vi "Edit Warning.vi"(7 "Warning in":string) -> (3 "Warning out":string)   [LabVIEW 2021, in "Converter.lvlib"]
uses:
  Converter.lvlib
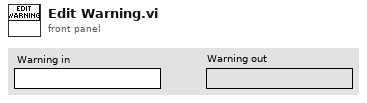
[diagram p1: front panel]
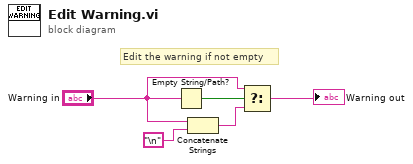
[diagram p0: block diagram]
diagram:
  # "Edit the warning if not empty"
  n1 = Empty String/Path?(string/path="Warning in") -> (empty?=w3:bool)
  n2 = Concatenate Strings("Warning in", "\n") -> (w5:string)
  n3 = Select(t="Warning in", s=w3, f=w5) -> (s? t:f=→"Warning out":string)
